vi "TreeSymbols.vi"(8 "error in (no error)":errorcluster, 10 "TreeControl in":refnum<vi>, 11 "ChannelsRepoBase in":refnum<class "ChannelsRepoXML.lvclass">) -> (0 "error out":errorcluster, 3 "ChannelsRepoBase out":refnum<class "ChannelsRepoXML.lvclass">)   [LabVIEW 2019]
doc: "Set the symbol for the AI AO DI DO channels in the tree"
uses:
  ChannelSettingsLib/ChannelsRepos/ChannelsRepoXML/ChannelsRepoXML.lvclass
  <vilib>/Bytelabs/{Package_File_Name}/Source/ByTree.lvlib
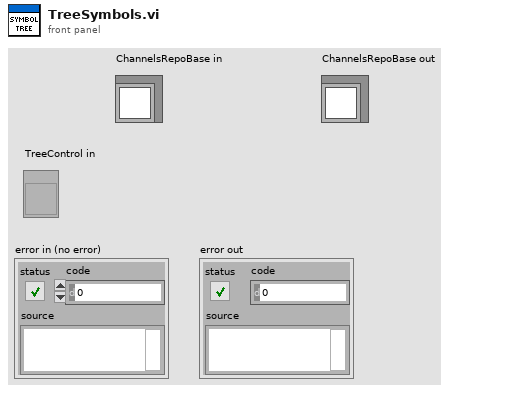
[diagram p1: front panel]
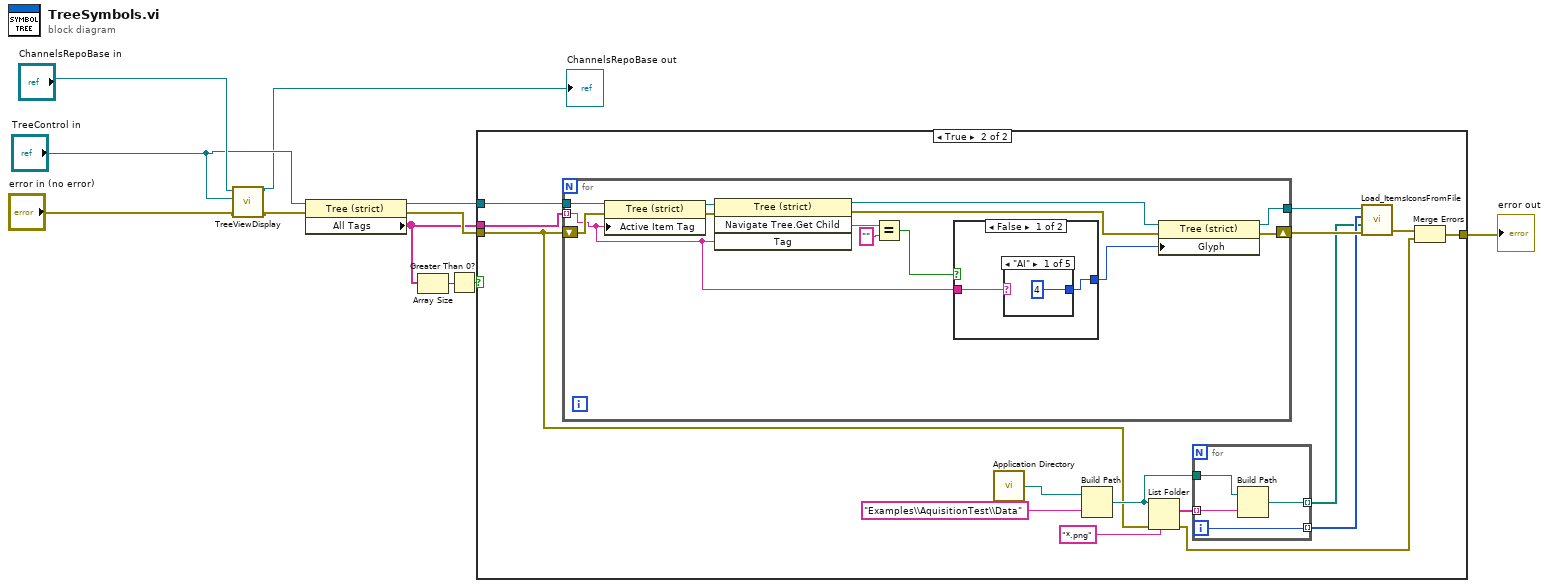
[diagram p0: block diagram]
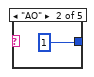
[diagram p3: hidden frame]
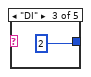
[diagram p4: hidden frame]
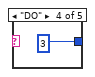
[diagram p5: hidden frame]
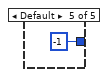
[diagram p6: hidden frame]
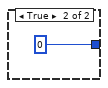
[diagram p7: hidden frame]
diagram:
  n1 = call-dynamic "TreeViewDisplay.vi"("error in (no error)"="error in (no error)", "Tree ref"="TreeControl in", "ChannelsRepoBase in"="ChannelsRepoBase in") -> ("error out"=w4:errorcluster, "ChannelsRepoBase out"=→"ChannelsRepoBase out":refnum<class "ChannelsRepoXML.lvclass">)  [unwired: 7 in]
  n2 = property class="Tree (strict)"(reference="TreeControl in", error in=w4) -> (reference out=w11:refnum<vi>, error out=w10:errorcluster, "All Tags"=w7:string[])
  n3 = Array Size(array=w7) -> (size(s)=w8:i32)
  n4 = Greater Than 0?(x=w8) -> (x > 0?=w6:bool)
  n5 = case shown="True" w6 {
    tunnel: w11 -> [_ w27]
    tunnel: w7 -> [_ w26]
    tunnel: w10 -> [w12 w16]
    tunnel: [w12 w14] -> w9
    frame False {
    }
    frame True {
      n6 = for {
        tunnel: w26 -> [w35] mode=indexing
        tunnel: w27 -> [w44]
        shift-right: [w33] -> w21
        shift-left: w16 -> [w43]
        tunnel: [w32] -> w20
        n7 = property class="Tree (strict)"(reference=w44, error in=w43, "Active Item Tag"=w35) -> (reference out=w42:refnum<vi>, error out=w38:errorcluster)
        n8 = invoke class="Tree (strict)" method="Navigate Tree.Get Child"(reference=w42, error in=w38, "Tag"=w35) -> (reference out=w41:refnum<vi>, error out=w34:errorcluster, "Navigate Tree:Get Child"=w40:string)  [unwired: 1 in, 1 out]
        n9 = Equal?(x=w40, y="") -> (x = y?=w37:bool)
        n10 = case shown="False" w37 {
          tunnel: [w45 0] -> w36
          tunnel: w35 -> [w46 _]
          frame False {
            n11 = case shown="\"AI\"" w46 {
              tunnel: [4 1 2 3 -1] -> w45
              frame "AI" {
              }
              frame "AO" {
              }
              frame "DI" {
              }
              frame "DO" {
              }
              frame Default {
              }
            }
          }
          frame True {
          }
        }
        n12 = property class="Tree (strict)"(reference=w41, error in=w34, "Glyph"=w36) -> (reference out=w32:refnum<vi>, error out=w33:errorcluster)
      }
      n13 = call <vilib>:"Application Directory.vi"() -> ("Application Directory"=w23:path)
      n14 = Build Path(base path=w23, name or relative path="Examples\\AquisitionTest\\Data") -> (appended path=w22:path)
      n15 = List Folder(path=w22, pattern="*.png", error in=w16) -> (filenames=w25:string[], error out=w13:errorcluster)  [unwired: 1 in, 2 out]
      n16 = for {
        tunnel: w25 -> [w31] mode=indexing
        tunnel: w22 -> [w30]
        tunnel: [w29] -> w18 mode=indexing
        tunnel: [w28] -> w19 mode=indexing
        i -> [w28]
        n17 = Build Path(base path=w30, name or relative path=w31) -> (appended path=w29:path)
      }
      n18 = call <vilib>:"Load_ItemsIconsFromFile.vi"("error in (no error)"=w21, "path to PNG file"=w18, "Index"=w19, "TreeControl in"=w20) -> ("error out"=w15:errorcluster)  [unwired: 6 in, 1 out]
      n19 = Merge Errors(w15, w13) -> (w14:errorcluster)
    }
  }
  "error out" <- w9
